vi "APT rotor sweep.vi"() -> ()   [LabVIEW 2012]
doc: "Shows how to move a motor to an absolute position."
uses:
  <vilib>/Math Plots/2D Math Plots/2D Compass/2D Compass XCtrl/2D Compass.xctl
  <vilib>/Analysis/1siggen.llb/Ramp Pattern by Samples.vi
  <vilib>/Utility/file.llb/Write To Spreadsheet File (DBL).vi
  <vilib>/Math Plots/2D Math Plots/2D Compass/2D Compass Datatype/Public/Plot Helper (Vector).vi
  <vilib>/Analysis/NI_AALBase.lvlib
  <vilib>/Math Plots/2D Math Plots/2D Compass/2D Compass Datatype/2D Compass Datatype.lvclass
panel:
  in  "track every":i32=3000
  in  "Y pos":dbl=122.0
  in  "X Pos":dbl=75.0
  in  "Y Parameters":T1={"Number of Y Steps"=200, "Max Y (V)"=2.0, "Min Y (V)"=-2.0}
  in  "X":T2={"Number of X Steps"=200, "Max X (V)"=2.0, "Min X (V)"=-2.0}
  in  "file path (dialog if empty)":path
  out "2D Compass":refnum<class "2D Plot Datatype.lvclass">[](xcontrol)
  out "XY Graph":cluster{"Y":dbl[], "Y":dbl[]}[](graph)
  in  "Time Target (s)":dbl=1.0
  in  "start":dbl format="%0.2f"
  in  "end":dbl=180.0 format="%0.2f"
  in  "samples":i32=90
  in  "MG17Motor":refnum<k7>(container)
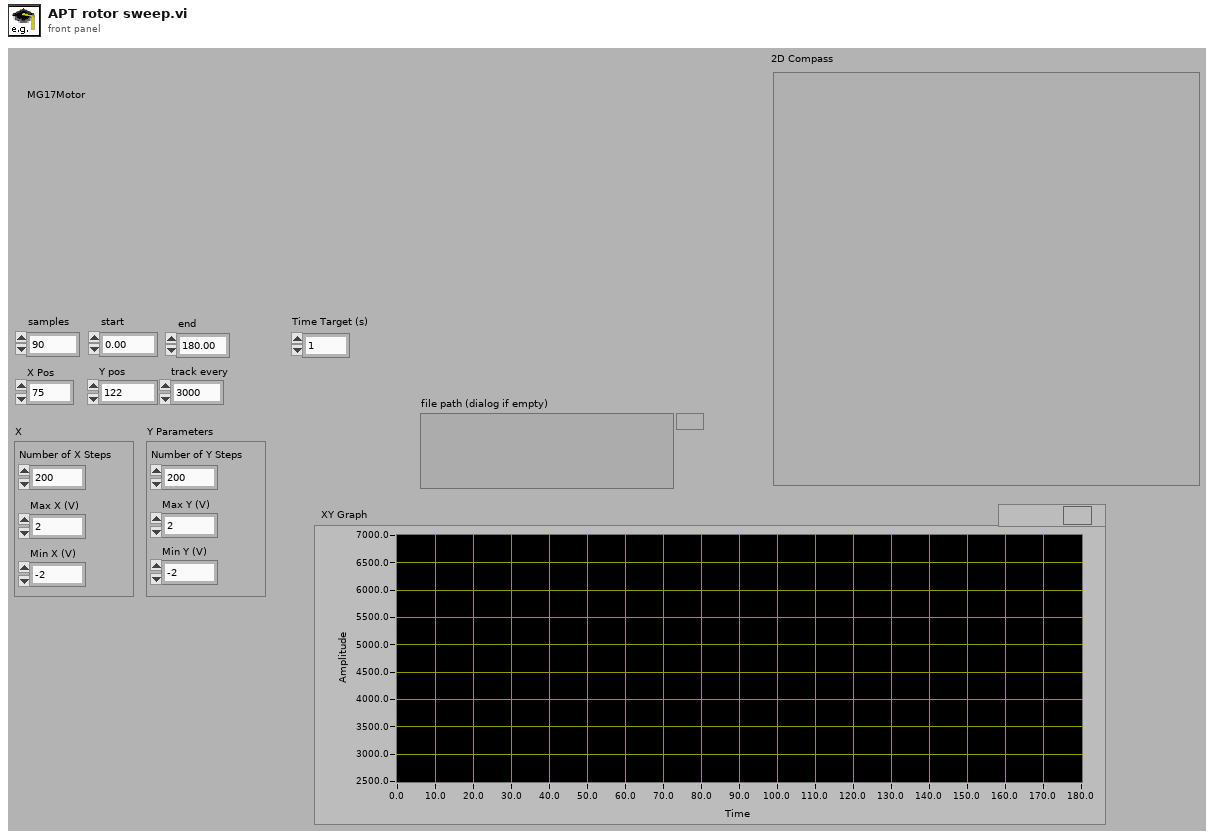
[diagram p1: front panel]
types:
  T1 = cluster{"Number of Y Steps":i32, "Max Y (V)":dbl, "Min Y (V)":dbl}
  T2 = cluster{"Number of X Steps":i32, "Max X (V)":dbl, "Min X (V)":dbl}
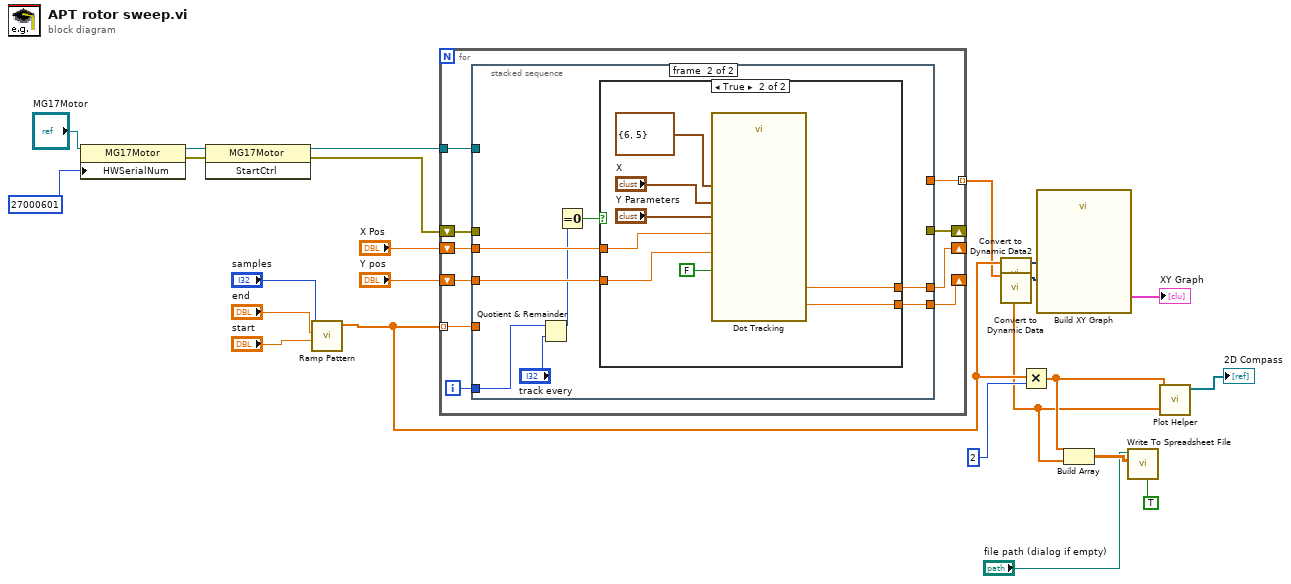
[diagram p0: block diagram]
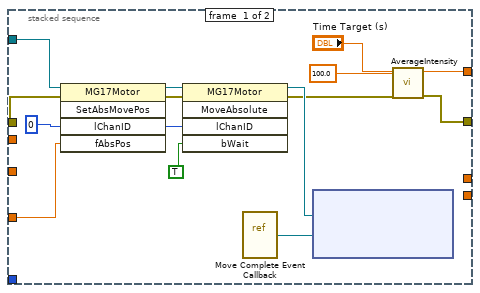
[diagram p2: hidden frame]
diagram:
  n1 = property class="MG17Motor"(reference="MG17Motor", "HWSerialNum"=27000601) -> (reference out=w21:refnum<k7>, error out=w19:errorcluster)  [unwired: 1 in]
  n2 = invoke class="MG17Motor" method="StartCtrl"(reference=w21, error in=w19) -> (reference out=w15:refnum<k7>, error out=w14:errorcluster)  [unwired: 1 in, 1 out]
  n3 = call-poly <vilib>:"Ramp Pattern.vi"("start"="start", "end"="end", "samples"="samples") -> ("Ramp Pattern"=w8:dbl[])  [unwired: 7 in, 1 out]
  n4 = for {
    shift-left: w14 -> [w31]
    shift-right: [w29] -> _
    tunnel: w8 -> [w30] mode=indexing
    tunnel: w15 -> [w32]
    tunnel: [w28] -> w6 mode=indexing
    shift-right: [w25] -> _
    shift-left: "X Pos" -> [w27]
    shift-right: [w24] -> _
    shift-left: "Y pos" -> [w26]
    i -> [w23]
    n5 = stacked-sequence {
      tunnel: w32 -> [w46 _]
      tunnel: w31 -> [w45 _]
      tunnel: w30 -> [w38 _]
      tunnel: [w34 _] -> w29
      tunnel: [w33 _] -> w28
      tunnel: w27 -> [_ w54]
      tunnel: w26 -> [_ w53]
      tunnel: [_ w52] -> w25
      tunnel: [_ w51] -> w24
      tunnel: w23 -> [_ w50]
      frame #0 {
        w42 = 0 ("lChanID")
        n6 = invoke class="MG17Motor" method="SetAbsMovePos"(reference=w46, error in=w45, "lChanID"=w42, "fAbsPos"=w38) -> (reference out=w44:refnum<k7>, error out=w43:errorcluster)  [unwired: 1 in, 3 out]
        n7 = invoke class="MG17Motor" method="MoveAbsolute"(reference=w44, error in=w43, "lChanID"=w42, "bWait"=TRUE) -> (reference out=w41:refnum<k7>, error out=w37:errorcluster)  [unwired: 1 in, 3 out]
        n8 = vi-ref "Move Complete Event Callback.vi"() -> ("vi reference"=w40:refnum<vi>)
        n9 = node(w41, w40) -> ()  [unwired: 3 in, 2 out]
        n10 = call "AverageIntensity.vi"("error in"=w37, "rate (Hz)"=100.0, "Time Target (s)"="Time Target (s)") -> ("error out"=w34:errorcluster, "Average intensity (cts/s)"=w33:dbl)  [unwired: 7 in]
      }
      frame #1 {
        n11 = Quotient & Remainder(x=w50, y="track every") -> (x-y*floor(x/y)=w48:i32)  [unwired: 1 out]
        n12 = Equal To 0?(x=w48) -> (x = 0?=w47:bool)
        n13 = case shown="True" w47 {
          tunnel: w54 -> [w56 w61]
          tunnel: w53 -> [w55 w60]
          tunnel: [w56 w59] -> w52
          tunnel: [w55 w58] -> w51
          frame False {
          }
          frame True {
            n14 = call "Dot Tracking.vi"("X"="X", "Y Parameters"="Y Parameters", "RS232 settings"=cluster{"Portnumber":i32, "Baudrate":u16} {"Portnumber"=6, "Baudrate"=5}, "X Pos"=w61, "Y pos"=w60, "Z-track?"=FALSE) -> ("X Position"=w59:dbl, "Y Position"=w58:dbl)  [unwired: 3 in, 5 out]
          }
        }
      }
    }
  }
  n15 = call "Convert to Dynamic Data2"("Array"=w8) -> ("Dynamic Data Type"=w11:dynamicdata)  [unwired: 3 in]
  n16 = call "Convert to Dynamic Data"("Array"=w6) -> ("Dynamic Data Type"=w12:dynamicdata)  [unwired: 3 in]
  n17 = Multiply(x=w8, y=2) -> (x*y=w7:dbl[])
  n18 = call "Build XY Graph"("Y Input"=w12, "X Input"=w11) -> ("XY Graph"=→"XY Graph":cluster{"Y":dbl[], "Y":dbl[]}[])  [unwired: 3 in, 6 out]
  n19 = Build Array(w7, w6) -> (w5:dbl[][])
  n20 = call-poly <vilib>:"Write To Spreadsheet File.vi"("transpose? (no:F)"=TRUE, "2D data"=w5, "file path (dialog if empty)"="file path (dialog if empty)") -> ()  [unwired: 5 in, 1 out]
  n21 = call-poly <vilib>:"Plot Helper.vi"("radius vector"=w6, "theta vector"=w7) -> ("2D Plot Class Obj Array out"=→"2D Compass":refnum<class "2D Plot Datatype.lvclass">[])  [unwired: 2 in, 7 out]
